vi "Write condtional.vi"(5 "condtional":bool, 9 "LoopTunnel in":refnum<class "LoopTunnel.lvclass">) -> (3 "LoopTunnel out":refnum<class "LoopTunnel.lvclass">)   [LabVIEW 2014, in "Raspberry Pi Compatible Compiler for LabVIEW.lvlib" / "LoopTunnel.lvclass"]
uses:
  LoopTunnel.lvclass
  LoopTunnel.lvclass/LoopTunnel.ctl
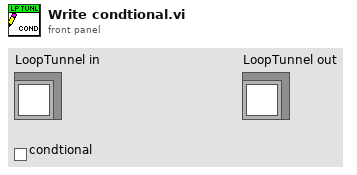
[diagram p1: front panel]
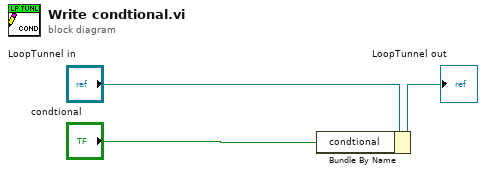
[diagram p0: block diagram]
diagram:
  n1 = Bundle By Name(cluster="LoopTunnel in", "condtional"="condtional") -> (→"LoopTunnel out":refnum<class "LoopTunnel.lvclass">)
